vi "Configure Analyzer Trigger.vi"(0 "VISA resource name":refnum<visa-resource-name>, 1 "Jitter Level (0 %FS)":i32, 2 "Trigger Polarity (0: trgRising)":u16(ring) items=["trgRising", "trgFalling"], 5 "Analyzer (0: A0)":i32(ring) items=["A0", "A1"], 7 "Enable Trigger (T: Enable)":bool=TRUE, 9 "Trigger Source (0: trgInputCh)":i32(ring) items=["trgInputCh", "trgOtherCh", "trgExt", "trgManual", "trgGen", "trgDigAudBlock", "trgBurstA", "trgBurstB"], 11 "error in (no error)":errorcluster, 12 "Generator Trigger Source (0: trgAnlgA)":i32(ring) items=["trgAnlgA", "trgAnlgB", "trgDigA", "trgDigB", "trgJitter"]) -> (4 "VISA resource name out":refnum<visa-resource-name>, 15 "error out":errorcluster)   [LabVIEW 2014, in "Stanford Research SR1.lvlib"]
doc: "Configures the Analyzer Trigger settings."
uses:
  Stanford Research SR1.lvlib
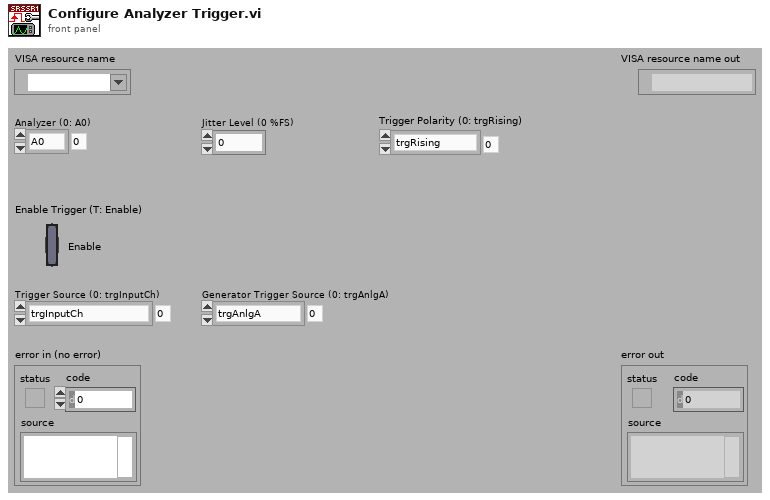
[diagram p1: front panel]
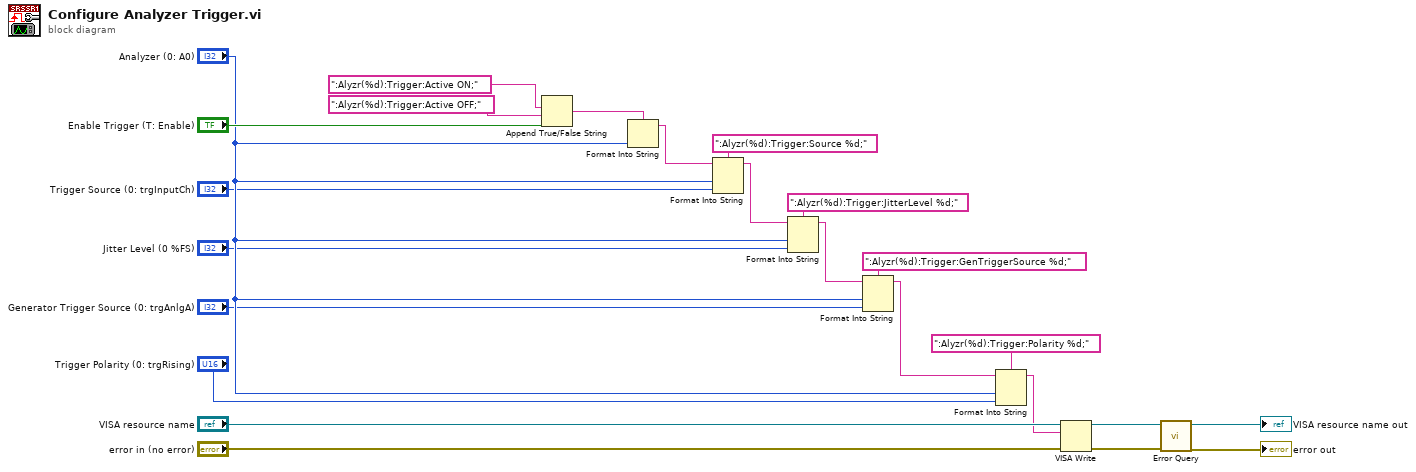
[diagram p0: block diagram]
diagram:
  n1 = Append True/False String(1:"Enable Trigger (T: Enable)", 2:":Alyzr(%d):Trigger:Active OFF;", 3:":Alyzr(%d):Trigger:Active ON;") -> (0:w10:string)  [unwired: 1 in]
  n2 = Format Into String(format string=w10, "Analyzer (0: A0)") -> (resulting string=w8:string)  [unwired: 2 in, 1 out]
  n3 = Format Into String(format string=":Alyzr(%d):Trigger:Source %d;", initial string=w8, "Analyzer (0: A0)", "Trigger Source (0: trgInputCh)") -> (resulting string=w20:string)  [unwired: 1 in, 1 out]
  n4 = Format Into String(format string=":Alyzr(%d):Trigger:JitterLevel %d;", initial string=w20, "Analyzer (0: A0)", "Jitter Level (0 %FS)") -> (resulting string=w18:string)  [unwired: 1 in, 1 out]
  n5 = Format Into String(format string=":Alyzr(%d):Trigger:GenTriggerSource %d;", initial string=w18, "Analyzer (0: A0)", "Generator Trigger Source (0: trgAnlgA)") -> (resulting string=w2:string)  [unwired: 1 in, 1 out]
  n6 = Format Into String(format string=":Alyzr(%d):Trigger:Polarity %d;", initial string=w2, "Analyzer (0: A0)", "Trigger Polarity (0: trgRising)") -> (resulting string=w4:string)  [unwired: 1 in, 1 out]
  n7 = VISA Write(VISA resource name="VISA resource name", write buffer=w4, error in (no error)="error in (no error)") -> (VISA resource name out=w14:refnum<visa-resource-name>, error out=w13:errorcluster)  [unwired: 1 out]
  n8 = call "Error Query.vi"("error in (no error)"=w13, "VISA resource name"=w14) -> ("error out"=→"error out":errorcluster, "VISA resource name out"=→"VISA resource name out":refnum<visa-resource-name>)  [unwired: 6 in, 2 out]
